vi "FTW-CodeGen-GetErrors.vi"(0 "State In":T2, 5 "XRef":refnum<vi>, 7 "Generate Strings?":bool) -> (4 "Errors":T1(array[cluster]), 6 "Errors Present?":bool)   [LabVIEW 2015, in "FTW-Array-Shuffle.xnode"]
uses:
  FTW-Array-Shuffle.xnode
  FTW-CodeGen-State.ctl
panel:
  # "Inputs"
  # "Outputs"
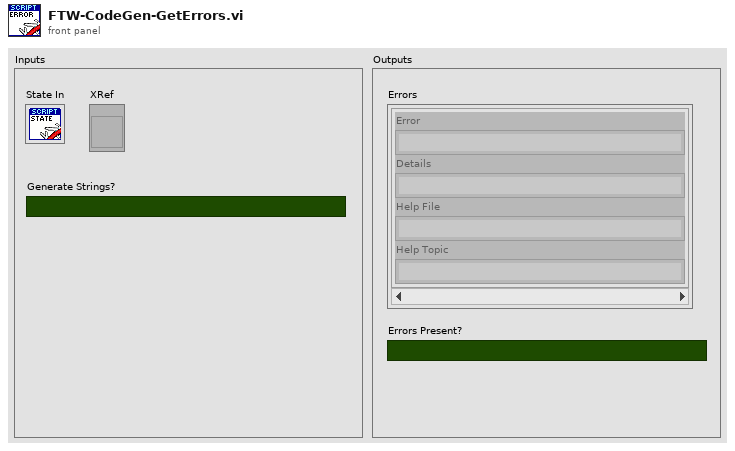
[diagram p1: front panel]
types:
  T1 = cluster{"Error":string, "Details":string, "Help File":string, "Help Topic":string}[]
  T2 = typedef "FTW-Array-Shuffle.xnode/FTW-CodeGen-State.ctl" = cluster{"Dummy":string}
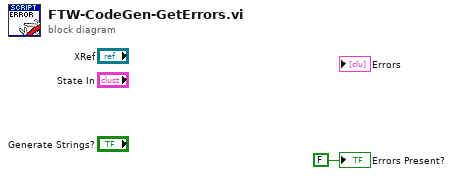
[diagram p0: block diagram]
diagram:
  "Errors Present?" <- FALSE ("Generated Code?")
